vi "Set Frequency Correction Value.vi"(8 "error in (no error)":errorcluster, 10 "Frequency Correction (ppm)":i32, 11 "DeviceRefnum":u64) -> (0 "error out":errorcluster, 2 "function return":i32, 3 "DeviceRefnum Out":u64)   [LabVIEW 2016]
doc: "Set the frequency correction value for the device."
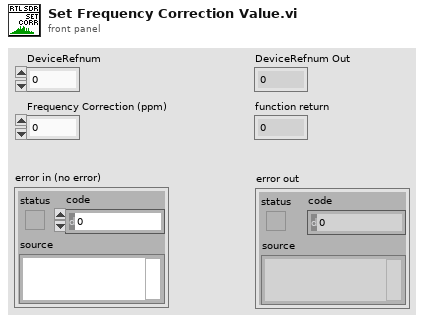
[diagram p1: front panel]
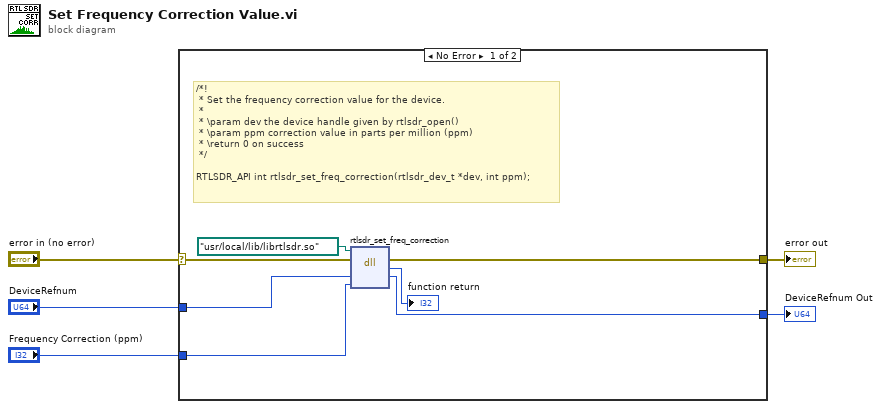
[diagram p0: block diagram]
diagram:
  n1 = case shown="No Error" "error in (no error)" {
    selector: "error in (no error)" -> [w6 w13]
    tunnel: [w11 w13] -> w5
    tunnel: "DeviceRefnum" -> [w10 w14]
    tunnel: "Frequency Correction (ppm)" -> [w9 _]
    tunnel: [w8 w14] -> w2
    frame No Error {
      # "/*!\n * Set the frequency correction value for the device.\n *\n * \\param dev the device handle given by rtlsdr_open()\n * \\param ppm correction value in parts per million (ppm)\n * \\return 0 on success\n */\n\nRTLSDR_API int rtlsdr_set_freq_correction(rtlsdr_dev_t *dev, int ppm);"
      n2 = dll-call lib="C:/Program Files (x86)/National Instruments/LabVIEW 2016/user.lib/rtlsdr/rtlsdr.*" fn="rtlsdr_set_freq_correction"(path in=path "/usr/local/lib/librtlsdr.so", error in=w6, "DeviceRefnum"=w10, "Frequency Correction (ppm)"=w9) -> (error out=w11:errorcluster, "return type"=→"function return":i32, "DeviceRefnum"=w8:u64)  [unwired: 2 in, 1 out]
    }
    frame Error {
    }
  }
  "error out" <- w5
  "DeviceRefnum Out" <- w2
